vi "rotate(NORMALNOE ROTATE).vi"(7 "On/Off\nRight/Left":bool, 8 "error in (no error)":errorcluster) -> (0 "error out":errorcluster)   [LabVIEW 2017]
uses:
  <vilib>/myRIO/Instrument Drivers/Onboard IO/I2C/typedefs/I2C Reference.ctl
  <vilib>/myRIO/Common/Instrument Driver Framework/Utilities/typedefs/myRIO Generic Hardware Reference.ctl
  <vilib>/myRIO/Common/Instrument Driver Framework/Utilities/typedefs/Hardware Version Enum.ctl
  <vilib>/myRIO/Common/Instrument Driver Framework/Utilities/typedefs/myRIO v1.0 Reference.ctl
  <vilib>/myRIO/Common/Instrument Driver Framework/Utilities/typedefs/Generic FPGA Reference.ctl
  <vilib>/myRIO/Common/Instrument Driver Framework/myRIO v1.0/I2C/typedefs/I2C Channels Enum.ctl
  <vilib>/myRIO/Instrument Drivers/Onboard IO/I2C/typedefs/I2C Configuration.ctl
  <vilib>/myRIO/Instrument Drivers/Onboard IO/I2C/typedefs/I2C Transfer Rate.ctl
  <vilib>/userdefined/High Color/nirio_resource_hc.ctl
  <vilib>/myRIO/Common/Instrument Driver Framework/myRIO v1.0/Encoder/typedefs/Encoder Signal Mode.ctl
  <vilib>/myRIO/Instrument Drivers/Onboard IO/Encoder/typedefs/Encoder Reference.ctl
  <vilib>/myRIO/Common/Instrument Driver Framework/myRIO v1.0/Encoder/typedefs/Encoder Channels Enum.ctl
  <vilib>/myRIO/Common/Instrument Driver Framework/myRIO v1.0/Encoder/typedefs/Encoder Configuration v1.0.ctl
  <vilib>/myRIO/Common/Instrument Driver Framework/myRIO v1.0/I2C/vis/myRIO v1.1 Open I2C.vi
  <vilib>/myRIO/Common/Instrument Driver Framework/Utilities/vis/Is FPGA Ref Available.vi
  <vilib>/myRIO/Common/Instrument Driver Framework/myRIO v1.0/Encoder/vis/myRIO v1.1 Open Encoder.vi
  <vilib>/myRIO/Instrument Drivers/Onboard IO/Encoder/vis/Read.vi
  <vilib>/myRIO/Common/Instrument Driver Framework/Utilities/vis/Validate Channels.vi
  <vilib>/myRIO/Common/Instrument Driver Framework/myRIO v1.0/I2C/vis/myRIO v1.0 Reserve I2C.vi
  <vilib>/myRIO/Common/Instrument Driver Framework/myRIO v1.0/Encoder/vis/myRIO v1.0 Reserve Encoder.vi
  <vilib>/myRIO/Common/Instrument Driver Framework/myRIO v1.0/I2C/vis/myRIO v1.0 Close I2C.vi
  <vilib>/myRIO/Common/Instrument Driver Framework/myRIO v1.0/I2C/vis/myRIO v1.0 Build MUX Configuration I2C.vi
  <vilib>/myRIO/Common/Instrument Driver Framework/myRIO v1.0/Resource Manager/vis/myRIO v1.0 Reserve Channel List.vi
  <vilib>/myRIO/Common/Instrument Driver Framework/myRIO v1.0/Encoder/vis/myRIO v1.0 Build MUX Configuration Encoder.vi
  <vilib>/myRIO/Common/Instrument Driver Framework/myRIO v1.0/I2C/vis/myRIO v1.0 Unreserve I2C.vi
  <vilib>/myRIO/Common/Instrument Driver Framework/myRIO v1.0/Resource Manager/vis/myRIO v1.0 Create Configuration List.vi
  <vilib>/myRIO/Common/Instrument Driver Framework/myRIO v1.0/Resource Manager/vis/myRIO v1.0 Reserve Channel.vi
  <vilib>/myRIO/Common/Instrument Driver Framework/myRIO v1.0/Resource Manager/vis/myRIO v1.0 Unreserve Channel.vi
  <vilib>/myRIO/Common/Instrument Driver Framework/myRIO v1.0/Resource Manager/vis/myRIO v1.0 Unreserve Channel List.vi
  <vilib>/myRIO/Common/Instrument Driver Framework/myRIO v1.0/Resource Manager/vis/myRIO v1.0 Build Mutex Name.vi
  <vilib>/Utility/VariantDataType/GetNumericInfo.vi
  <vilib>/Utility/error.llb/Error Cluster From Error Code.vi
  <vilib>/myRIO/Common/Instrument Driver Framework/myRIO v1.0/myRIO v1.1 Open.vi
  <vilib>/myRIO/Common/Instrument Driver Framework/Utilities/vis/IO Manager.vi
  <vilib>/myRIO/Common/Instrument Driver Framework/Utilities/vis/Configuration Manager.vi
  <vilib>/myRIO/Common/Instrument Driver Framework/myRIO v1.0/Resource Manager/vis/myRIO v1.0 Configure IO.vi
  <vilib>/myRIO/Common/Instrument Driver Framework/myRIO v1.0/myRIO v1.0 Close.vi
  <vilib>/myRIO/Common/Instrument Driver Framework/myRIO v1.0/Encoder/vis/myRIO v1.0 Configure Encoder.vi
  <vilib>/myRIO/Common/Instrument Driver Framework/myRIO v1.0/Encoder/vis/myRIO v1.0 Read Encoder.vi
  <vilib>/imath/engines/lvmath2/RunTimeEngine/Managers/WorkSpace/UID Generator.vi
  <vilib>/imath/engines/lvmath2/RunTimeEngine/RunTimeType/NIMS_RunTimeType_From StrictType (excl LVString).vi
  <instcachedir>/0/NIMS_RunTimeType_From StrictType (excl LVString)_1019F277F0A747EDBCA0F6C52CA54500.lvgen/NIMS_RunTimeType_From StrictType (excl LVString)_1019F277F0A747EDBCA0F6C52CA54500_000.vi
  <vilib>/imath/engines/lvmath2/RunTimeEngine/LocalVariableDefStatement/MC_LocalVariableDefStatement_Display.vi
  <vilib>/imath/engines/lvmath2/RunTimeEngine/Managers/SymbolTable/Clear UID.vi
  <vilib>/imath/engines/lvmath2/RunTimeEngine/NodeEndStatement/NIMS_NodeEndStatement_Output.vi
  <instcachedir>/0/NIMS_NodeEndStatement_Output_53EC0D466D134D7ABD903AC30B43404B.lvgen/NIMS_NodeEndStatement_Output_53EC0D466D134D7ABD903AC30B43404B_013.vi
  <vilib>/imath/engines/lvmath2/RunTimeEngine/ErrorHandling/NIMS_Finalize Error.vi
  <vilib>/myRIO/Common/Instrument Driver Framework/myRIO v1.0/DIO/vis/myRIO v1.0 Write DIO.vi
  <vilib>/myRIO/Common/Instrument Driver Framework/myRIO v1.0/I2C/vis/myRIO v1.0 Shutdown I2C.vi
  <vilib>/myRIO/Instrument Drivers/Onboard IO/I2C/vis/myRIO I2C Open.xnode
  <vilib>/myRIO/Express VI/Onboard IO/Encoder/Encoder Express VI.xnode
  <vilib>/myRIO/Instrument Drivers/Onboard IO/Encoder/vis/myRIO Encoder Open.xnode
  <vilib>/myRIO/Common/Instrument Driver Framework/myRIO v1.0/Encoder/typedefs/Encoder Count Direction Enum.ctl
  <vilib>/myRIO/Instrument Drivers/Onboard IO/I2C/I2C.lvlib
  <vilib>/myRIO/Instrument Drivers/Onboard IO/Encoder/Encoder.lvlib
  <vilib>/imath/engines/lvmath2/RunTimeEngine/Managers/SymbolTable/NIMS_WorkSpace.lvlib
  <vilib>/myRIO/Instrument Drivers/Onboard IO/DIO/DIO.lvlib
panel:
  out "angle Z(coerset)":ext
  out "main angle":ext
  out "angle Z":ext
  out "zMax right":ext
  out "zMin right":ext
  in  "Stop Motor(true block)":bool
  out "zMin left":ext
  out "zMax left":ext
  in  "Stop Motor(false block)":bool
  in  "Stop Button":bool
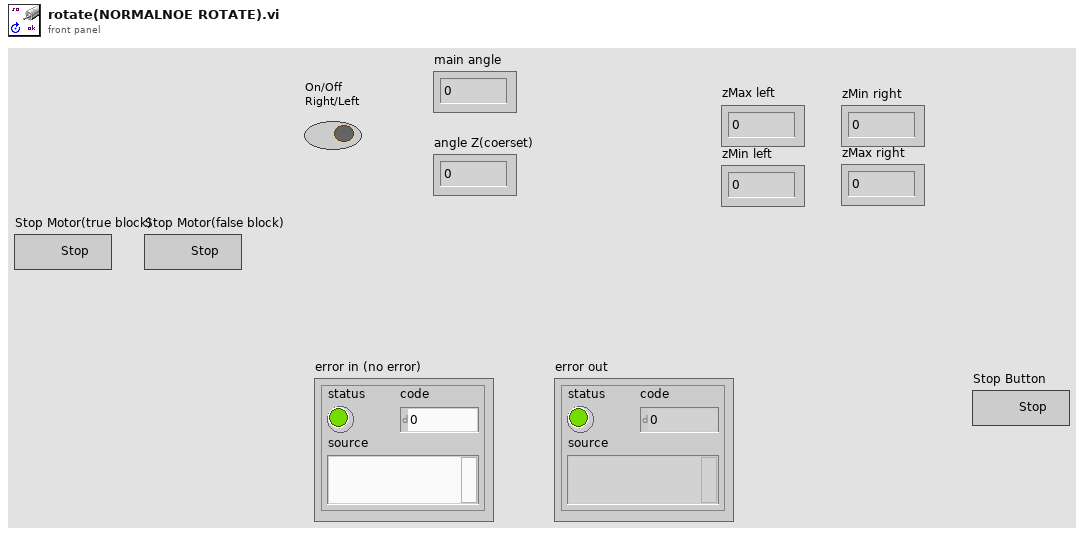
[diagram p1: front panel]
types:
  T1 = typedef "I2C.lvlib/I2C Reference.ctl" = cluster{"myRIO Reference":T2, "I2C Channels Enum":T6, "I2C Configuration":T7}
  T2 = typedef "myRIO Generic Hardware Reference.ctl" = cluster{"myRIO Model":T3, "myRIO Hardware Reference":T4}
  T3 = typedef "Hardware Version Enum.ctl" = enum16{"Unknown", "myRIO-1900", "myRIO-1950", "roboRIO", "NI ELVIS RIO CM"}
  T4 = typedef "myRIO v1.0 Reference.ctl" = cluster{"Generic FPGA Reference":T5, "Allow multiple opens":bool}
  T5 = typedef "Generic FPGA Reference.ctl" = refnum<k20>
  T6 = typedef "I2C Channels Enum.ctl" = enum16{"Not Connected", "A/I2C", "B/I2C", "I2C/I2C"}
  T7 = typedef "I2C.lvlib/I2C Configuration.ctl" = cluster{"I2C Transfer Rate":T8}
  T8 = typedef "I2C.lvlib/I2C Transfer Rate.ctl" = enum16{"Standard mode (100 kbps)", "Fast mode (400 kbps)"}
  T9 = typedef "DIO.lvlib/DIO Reference.ctl" = cluster{"myRIO Reference":T2, "DIO Channels List":T10}
  T10 = typedef "DIO Channels List.ctl" = T11[]
  T11 = typedef "DIO Channels Enum.ctl" = enum16{"Not Connected", "C/DIO0", "C/DIO1", "C/DIO2", "C/DIO3", "C/DIO4", "C/DIO5", "C/DIO6", "C/DIO7", "A/DIO0", "A/DIO1", "A/DIO2", "A/DIO3", "A/DIO4", "A/DIO5", "A/DIO6", "A/DIO7", "A/DIO8", "A/DIO9", "A/DIO10", "A/DIO11", "A/DIO12", "A/DIO13", "A/DIO14", "A/DIO15", "B/DIO0", "B/DIO1", "B/DIO2", "B/DIO3", "B/DIO4", "B/DIO5", "B/DIO6", "B/DIO7", "B/DIO8", "B/DIO9", "B/DIO10", "B/DIO11", "B/DIO12", "B/DIO13", "B/DIO14", "B/DIO15", "LED0", "LED1", "LED2", "LED3", "Button0", "DIO/DIO0", "DIO/DIO1", "DIO/DIO2", "DIO/DIO3", "DIO/DIO4", "DIO/DIO5", "DIO/DIO6", "DIO/DIO7", "DIO/DIO8", "DIO/DIO9", "SPI/CS0", "SPI/CS1", "SPI/CS2", "SPI/CS3", "LED RADIO (Green)", "LED RADIO (Red)", "LED COMM (Green)", "LED COMM (Red)", "LED MODE (Green)", "LED MODE (Red)"}
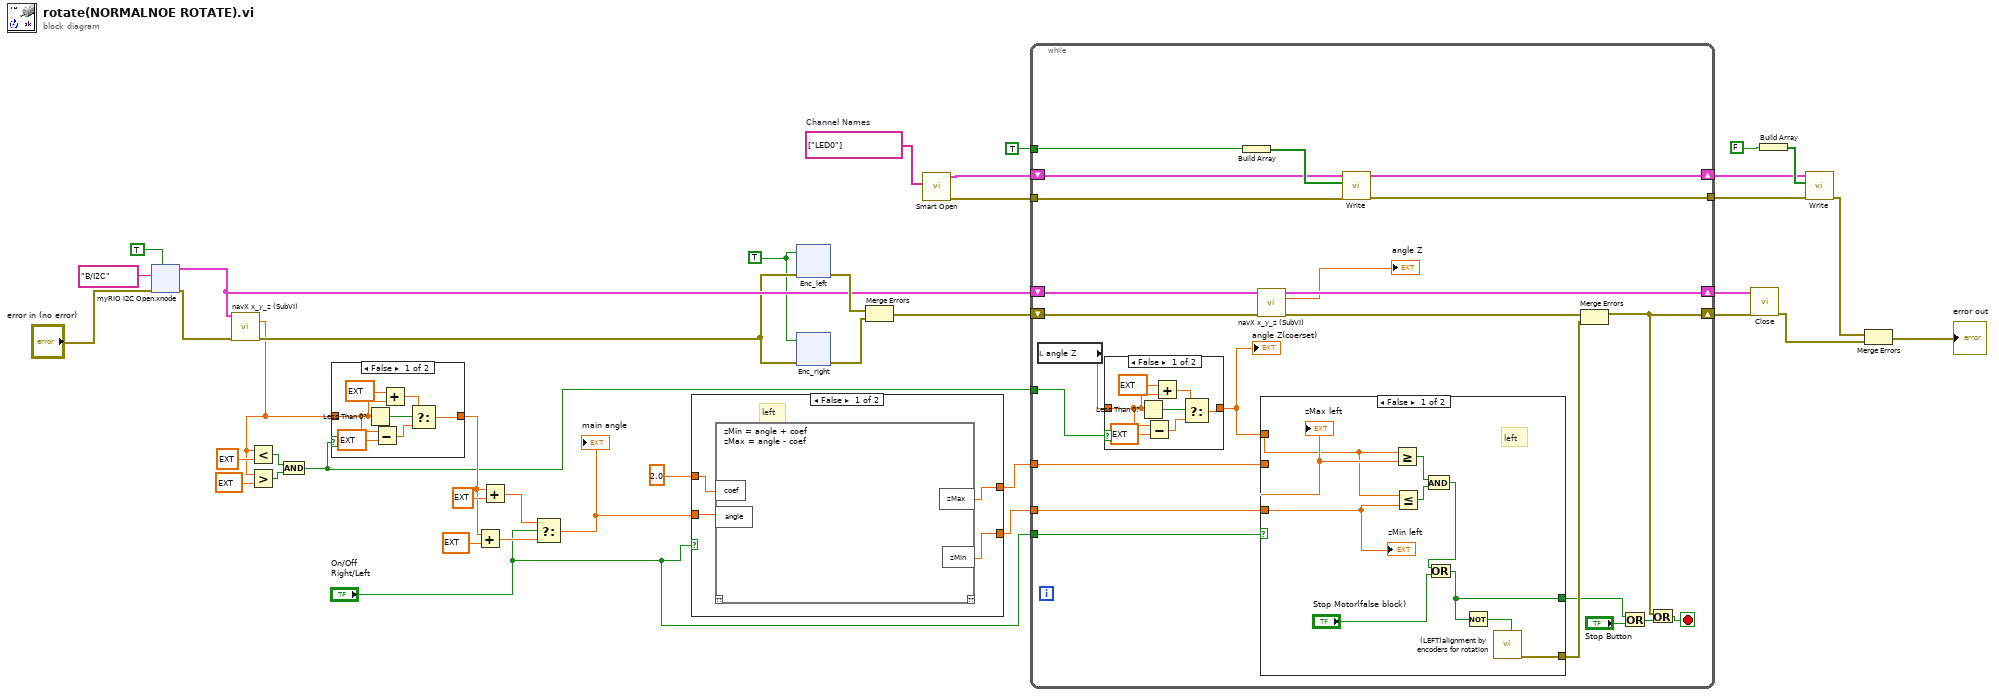
[diagram p0: block diagram]
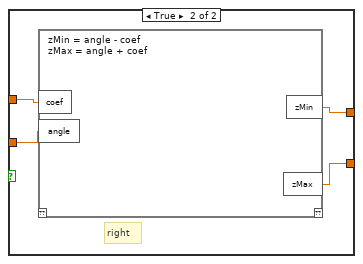
[diagram p3: hidden frame]
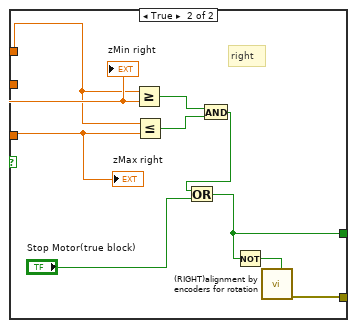
[diagram p5: hidden frame]
diagram:
  w10 = tag[] ["LED0"]  # Channel Names
  w23 = TRUE
  n1 = xnode "myRIO I2C Open.xnode"("error in (no error)"="error in (no error)", "Allow multiple opens?"=TRUE, "Channel Name"=tag "B/I2C") -> ("error out"=w25:errorcluster, "I2C Ref Out"=w32:T1)
  n2 = call "navX x_y_z (SubVI).vi"("I2C Ref Out in"=w32, "error in (no error)"=w25) -> ("value Z"=w11:ext, "error out"=w26:errorcluster)  [unwired: 9 in, 3 out]
  n3 = Less?(x=w11, y=ext 90.0) -> (x < y?=w15:bool)
  n4 = Greater?(x=w11, y=ext -90.0) -> (0:w17:bool)
  n5 = And(x=w15, y=w17) -> (x .and. y?=w12:bool)
  n6 = case shown="False" w12 {
    tunnel: [w45 w47] -> w13
    tunnel: w11 -> [w40 w47]
    frame False {
      n7 = Less Than 0?(x=w40) -> (x < 0?=w46:bool)
      n8 = Subtract(x=w40, y=ext 180.0) -> (x-y=w42:ext)
      n9 = Add(x=ext 180.0, y=w40) -> (x+y=w44:ext)
      n10 = Select(t=w44, s=w46, f=w42) -> (s? t:f=w45:ext)
    }
    frame True {
    }
  }
  n11 = Add(x=w13, y=ext -90.0) -> (x+y=w31:ext)
  n12 = Add(x=w13, y=ext 90.0) -> (x+y=w30:ext)
  n13 = Select(t=w30, s="On/Off\nRight/Left", f=w31) -> (s? t:f=w14:ext)
  "main angle" <- w14
  n14 = case shown="False" "On/Off\nRight/Left" {
    tunnel: 2.0 ("coef") -> [w51 w110]
    tunnel: w14 -> [w50 w109]
    tunnel: [w48 w108] -> w21
    tunnel: [w49 w107] -> w20
    frame False {
      # "left"
      n15 = mathscript code="zMin = angle + coef\nzMax = angle - coef"("angle"=w50, "coef"=w51) -> ("zMin"=w49:ext, "zMax"=w48:ext)  [unwired: 1 in, 1 out]
    }
    frame True {
      # "right"
      n16 = mathscript code="zMin = angle - coef\nzMax = angle + coef"("angle"=w109, "coef"=w110) -> ("zMin"=w108:ext, "zMax"=w107:ext)  [unwired: 1 in, 1 out]
    }
  }
  n17 = xnode "Enc_left"("error in (no error)"=w26, "Reset Counter"=w23) -> ("error out"=w34:errorcluster)  [unwired: 3 out]
  n18 = xnode "Enc_right"("error in (no error)"=w26, "Reset Counter"=w23) -> ("error out"=w33:errorcluster)  [unwired: 3 out]
  n19 = Merge Errors(w34, w33) -> (w39:errorcluster)
  n20 = call <vilib>:"Smart Open.vi"("Channel Names"=w10) -> ("error out"=w5:errorcluster, "DIO Ref Out"=w3:T9)  [unwired: 9 in]
  n21 = while {
    shift-right: [w176] -> w38
    shift-left: w39 -> [w187]
    tunnel: "On/Off\nRight/Left" -> [w184]
    shift-right: [w183] -> w35
    shift-left: w32 -> [w188]
    tunnel: w21 -> [w180]
    tunnel: w20 -> [w179]
    tunnel: w12 -> [w173]
    tunnel: w5 -> [w168]
    tunnel: [w167] -> w4
    shift-right: [w170] -> w6
    shift-left: w3 -> [w169]
    tunnel: TRUE -> [w166]
    stop <- w177 stop-if-true
    n22 = local read "angle Z"() -> (w172:ext)
    n23 = case shown="False" w173 {
      tunnel: [w194 w196] -> w174
      tunnel: w172 -> [w189 w196]
      frame False {
        n24 = Less Than 0?(x=w189) -> (x < 0?=w195:bool)
        n25 = Subtract(x=w189, y=ext 180.0) -> (x-y=w191:ext)
        n26 = Add(x=ext 180.0, y=w189) -> (x+y=w193:ext)
        n27 = Select(t=w193, s=w195, f=w191) -> (s? t:f=w194:ext)
      }
      frame True {
      }
    }
    "angle Z(coerset)" <- w174
    n28 = Build Array(w166) -> (w171:bool[])
    n29 = call "navX x_y_z (SubVI).vi"("I2C Ref Out in"=w188, "error in (no error)"=w187) -> ("I2C Ref Out out"=w183:T1, "value Z"=→"angle Z":ext, "error out"=w185:errorcluster)  [unwired: 9 in, 2 out]
    n30 = case shown="False" w184 {
      tunnel: [w200 w211] -> w181
      tunnel: [w204 w210] -> w186
      tunnel: w180 -> [w198 w208]
      tunnel: w179 -> [w199 w209]
      tunnel: w174 -> [w197 w207]
      frame False {
        # "left"
        n31 = Greater Or Equal?(x=w197, y=w198) -> (x >= y?=w205:bool)
        n32 = Less Or Equal?(x=w197, y=w199) -> (x <= y?=w206:bool)
        n33 = And(x=w205, y=w206) -> (x .and. y?=w203:bool)
        n34 = Or(x=w203, y="Stop Motor(false block)") -> (x .or. y?=w200:bool)
        n35 = Not(x=w200) -> (.not. x?=w201:bool)
        n36 = call "(LEFT)alignment by encoders for rotation.vi"("On/Off"=w201) -> ("error out"=w204:errorcluster)  [unwired: 10 in]
        "zMin left" <- w199
        "zMax left" <- w198
      }
      frame True {
        # "right"
        n37 = Greater Or Equal?(x=w207, y=w208) -> (x >= y?=w216:bool)
        n38 = Less Or Equal?(x=w207, y=w209) -> (x <= y?=w215:bool)
        n39 = And(x=w216, y=w215) -> (x .and. y?=w214:bool)
        n40 = Or(x=w214, y="Stop Motor(true block)") -> (x .or. y?=w211:bool)
        n41 = Not(x=w211) -> (.not. x?=w212:bool)
        n42 = call "(RIGHT)alignment by encoders for rotation.vi"("On/Off"=w212) -> ("error out"=w210:errorcluster)  [unwired: 10 in]
        "zMax right" <- w209
        "zMin right" <- w208
      }
    }
    n43 = call <vilib>:"Write.vi"("error in (no error)"=w168, "Values"=w171, "DIO Ref In"=w169) -> ("error out"=w167:errorcluster, "DIO Ref Out"=w170:T9)  [unwired: 6 in]
    n44 = Merge Errors(w185, w186) -> (w176:errorcluster)
    n45 = Or(x=w181, y="Stop Button") -> (x .or. y?=w178:bool)
    n46 = Or(x=w176, y=w178) -> (x .or. y?=w177:bool)
  }
  n47 = call <vilib>:"Close.vi"("error in (no error)"=w38, "I2C Ref In"=w35) -> ("error out"=w24:errorcluster)  [unwired: 9 in]
  n48 = Build Array(FALSE) -> (w9:bool[])
  n49 = call <vilib>:"Write.vi"("error in (no error)"=w4, "Values"=w9, "DIO Ref In"=w6) -> ("error out"=w7:errorcluster)  [unwired: 6 in, 1 out]
  n50 = Merge Errors(w7, w24) -> (→"error out":errorcluster)
